vi "Remove.vi"(8 "error in (no error)":errorcluster, 10 "Index":i32, 11 "Database Entry in":refnum<class "Database Entry.lvclass">) -> (0 "error out":errorcluster, 3 "Database Entry out":refnum<class "Database Entry.lvclass">)   [LabVIEW 2021, in "Database Entry.lvclass"]
uses:
  Database Entry.lvclass
  Database Entry.lvclass/Database Entry.ctl
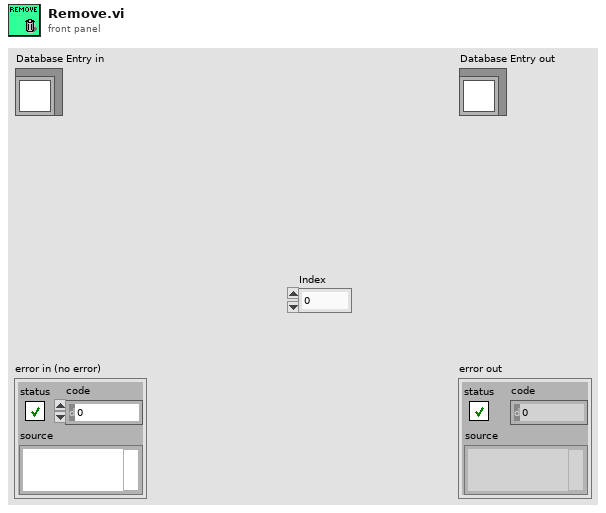
[diagram p1: front panel]
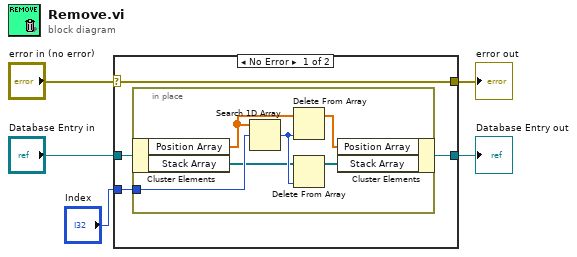
[diagram p0: block diagram]
diagram:
  n1 = case shown="No Error" "error in (no error)" {
    selector: "error in (no error)" -> [w9 w17]
    tunnel: [w9 w17] -> w4
    tunnel: [w6 w16] -> w3
    tunnel: "Database Entry in" -> [w7 w16]
    tunnel: "Index" -> [w8 _]
    frame No Error {
      n2 = in-place {
        in-place-border: w8 -> [w14]
        n3 = in-place-cluster #1(w7) -> ("Position Array"=w13:dbl[], "Stack Array"=w12:refnum<class "Stack.lvclass">[])
        n4 = Search 1D Array(1D array=w13, element=w14) -> (index of element=w15:i32)  [unwired: 1 in]
        n5 = Delete From Array(array=w13, index=w15) -> (array with subset deleted=w11:dbl[])  [unwired: 1 in, 1 out]
        n6 = Delete From Array(array=w12, index=w15) -> (array with subset deleted=w10:refnum<class "Stack.lvclass">[])  [unwired: 1 in, 1 out]
        n7 = in-place-cluster #1("Position Array"=w11, "Stack Array"=w10) -> (w6:refnum<class "Database Entry.lvclass">)
      }
    }
    frame Error {
    }
  }
  "error out" <- w4
  "Database Entry out" <- w3
